vi "Get FileGlobals.vi"(8 "error in (no error)":errorcluster, 11 "Session Handle in":T2) -> (0 "error out":errorcluster, 2 "FileGlobals":T1, 3 "Session Handle out":T2)   [LabVIEW 2020, in "TSS.lvlib" / "SequenceFile.lvclass"]
uses:
  SequenceFile.lvclass
  Typedefs/Session Handle.ctl
  VariableContainer/Typedefs/Session Handle.ctl
  VariableContainer/VariableContainer.lvclass
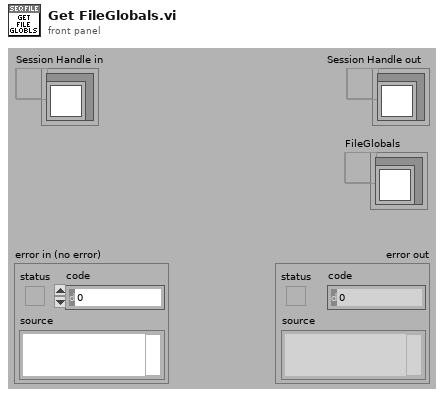
[diagram p1: front panel]
types:
  T1 = typedef "TSS.lvlib/VariableContainer.lvclass/Session Handle.ctl" = refnum<data-value>
  T2 = typedef "TSS.lvlib/SequenceFile.lvclass/Session Handle.ctl" = refnum<data-value>
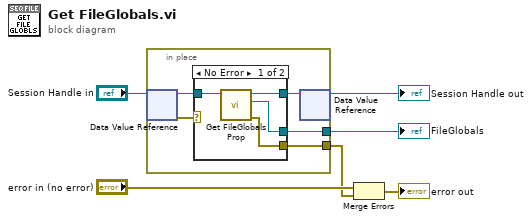
[diagram p0: block diagram]
diagram:
  n1 = in-place {
    in-place-border: [w9] -> w3
    in-place-border: [w7] -> w1
    n2 = in-place-dvr #1("Session Handle in") -> (w10:refnum<class "SequenceFile.lvclass">, w11:errorcluster)
    n3 = case shown="No Error" w11 {
      selector: w11 -> [_ w16]
      tunnel: w10 -> [w15 w17]
      tunnel: [w13 _] -> w9
      tunnel: [w14 w17] -> w8
      tunnel: [w12 w16] -> w7
      frame No Error {
        n4 = call "Get FileGlobals Prop.vi"("SequenceFile in"=w15) -> ("error out"=w12:errorcluster, "FileGlobals"=w13:T1, "SequenceFile out"=w14:refnum<class "SequenceFile.lvclass">)  [unwired: 8 in]
      }
      frame Error {
      }
    }
    n5 = in-place-dvr #1(w8) -> (→"Session Handle out":T2)  [unwired: 1 out]
  }
  "FileGlobals" <- w3
  n6 = Merge Errors("error in (no error)", w1) -> (→"error out":errorcluster)
